vi "Parallel VIs Launcher.vi"() -> ()   [LabVIEW 2013, in "TestVIs.lvlib"]
uses:
  TestVIs.lvlib
panel:
  out "Total Processes Still Running":i16
  out "Total Processes Successfully Launched":i16
  out "Total Processes Requested To Be Launched":i32
  in  "Desired Instances, per kind":i32=2
  # "This will launch a total of 10n + 5 processes"
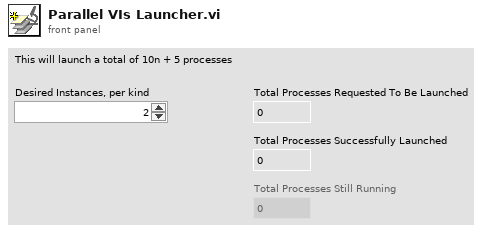
[diagram p1: front panel]
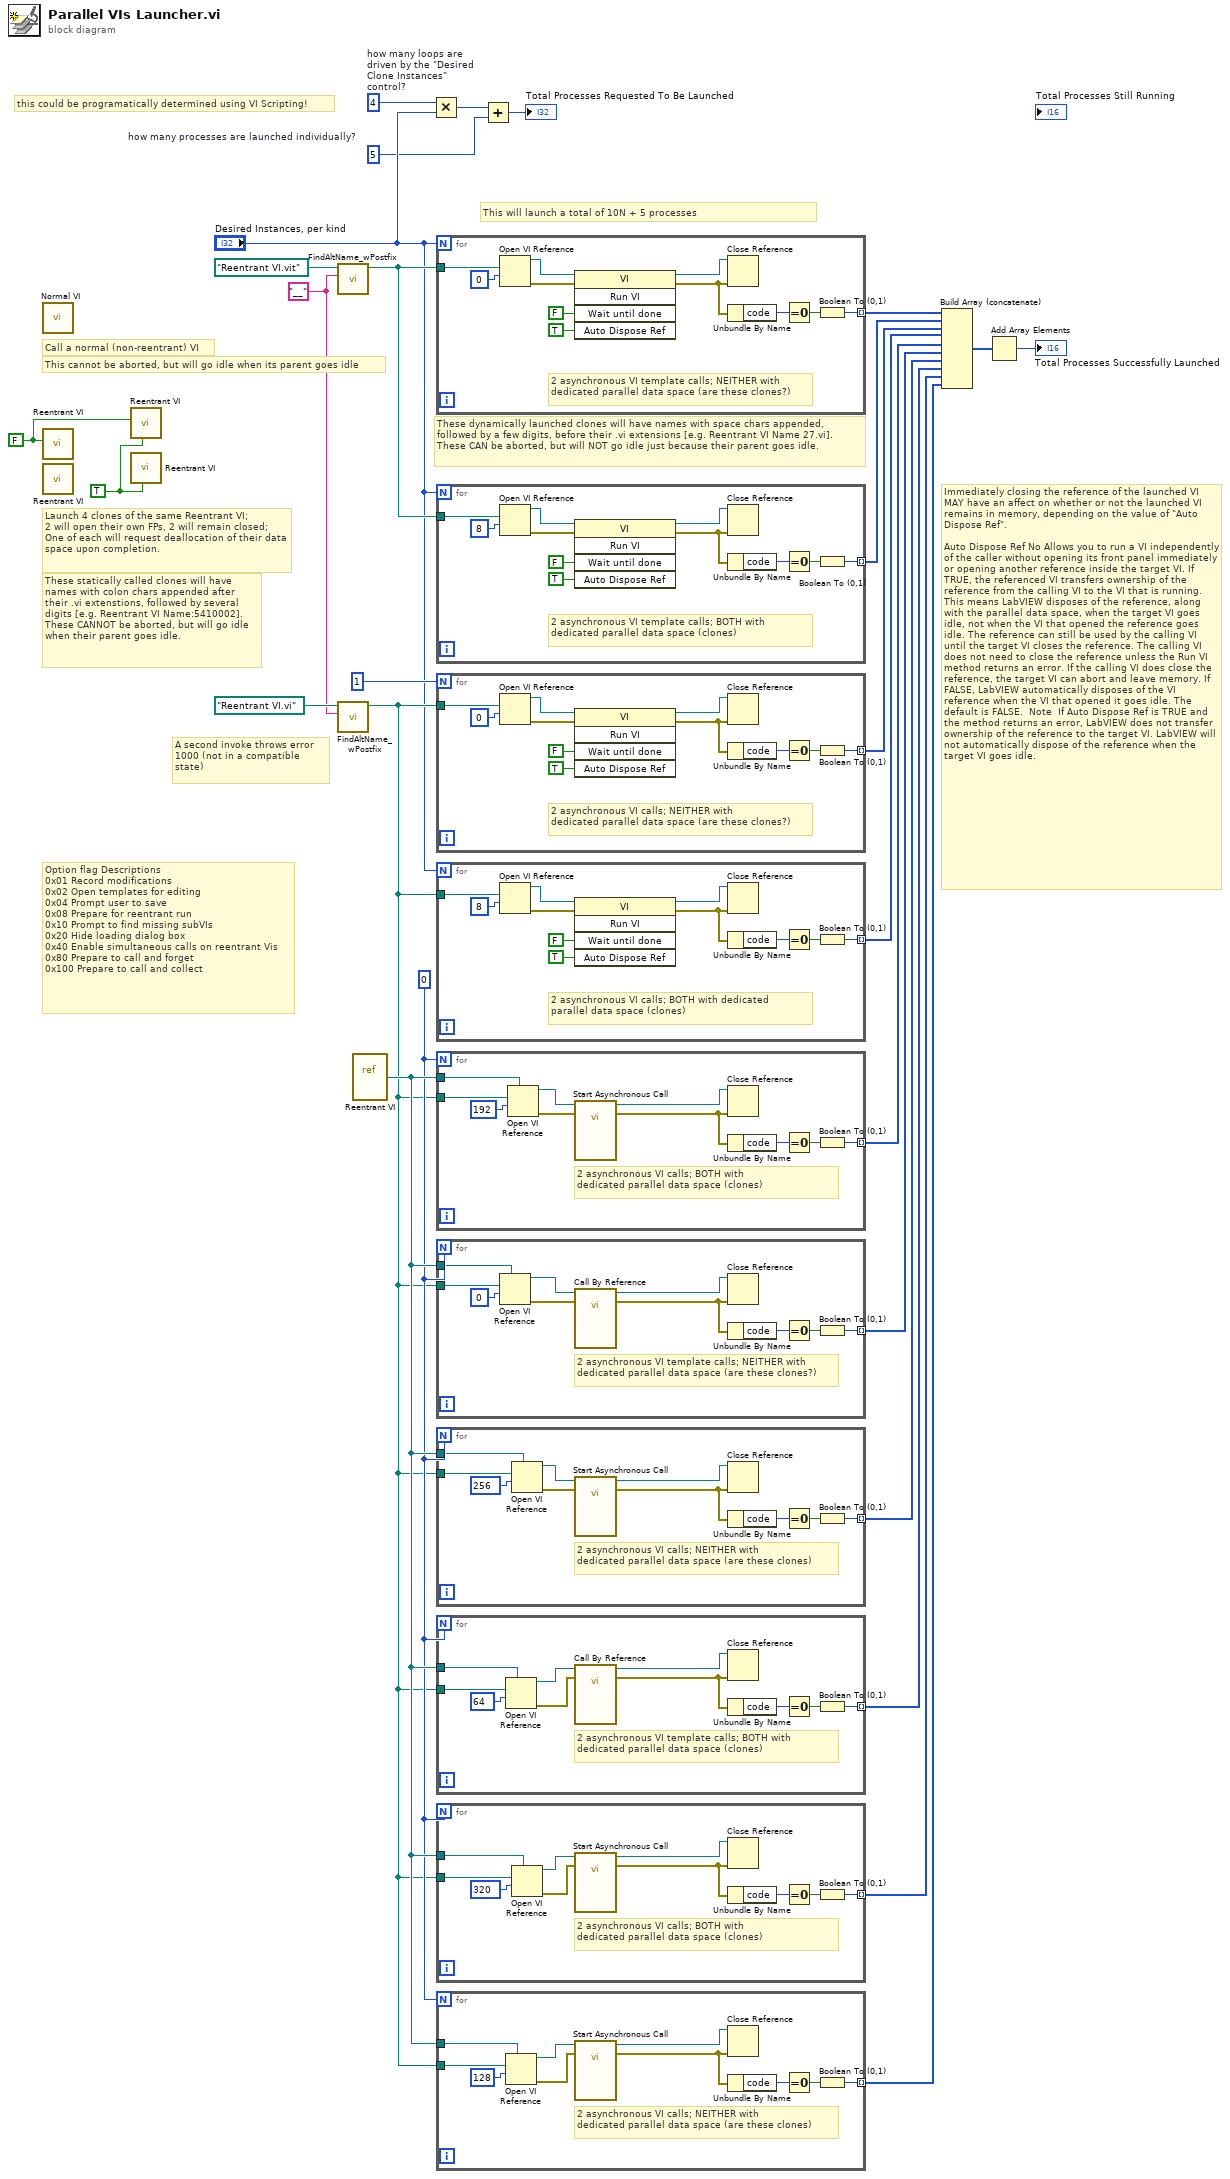
[diagram p0: block diagram]
diagram:
  w14 = 5  # how many processes are launched individually?
  w16 = 4  # how many loops are driven by the "Desired Clone Instances" control?
  w19 = "__" ("Token")
  w23 = 0
  w24 = TRUE ("Request Deallocation?")
  w22 = FALSE ("Open FP?")
  # "Immediately closing the reference of the launched VI MAY have an affect on whether or not the launched VI remains in memory, depending on the value of \"Auto Dispose Ref\".\n\nAuto Dispose Ref No Allows you to run a VI independently of the caller without opening its front panel immediately or opening another reference inside the target VI. If TRUE, the referenced VI transfers ownership of the reference from the calling VI to the VI that is running. This means LabVIEW disposes of the reference, along with the parallel data space, when the target VI goes idle, not when the VI that opened the reference goes idle. The reference can still be used by the calling VI until the target VI closes the reference. The calling VI does not need to close the reference unless the Run VI method returns an error. If the calling VI does close the reference, the target VI can abort and leave memory. If FALSE, LabVIEW automatically disposes of the VI reference when the VI that opened it goes idle. The default is FALSE.  Note  If Auto Dispose Ref is TRUE and the method returns an error, LabVIEW does not transfer ownership of the reference to the target VI. LabVIEW will not automatically dispose of the reference when the target VI goes idle."
  # "A second invoke throws error 1000 (not in a compatible state)"
  # "Option flag Descriptions \n0x01 Record modifications\n0x02 Open templates for editing\n0x04 Prompt user to save\n0x08 Prepare for reentrant run\n0x10 Prompt to find missing subVIs\n0x20 Hide loading dialog box\n0x40 Enable simultaneous calls on reentrant Vis\n0x80 Prepare to call and forget\n0x100 Prepare to call and collect"
  # "this could be programatically determined using VI Scripting!"
  # "These dynamically launched clones will have names with space chars appended, followed by a few digits, before their .vi extensions [e.g. Reentrant VI Name 27.vi].\nThese CAN be aborted, but will NOT go idle just because their parent goes idle."
  # "These statically called clones will have names with colon chars appended after their .vi extenstions, followed by several digits [e.g. Reentrant VI Name:5410002].\nThese CANNOT be aborted, but will go idle when their parent goes idle."
  # "This cannot be aborted, but will go idle when its parent goes idle"
  # "This will launch a total of 10N + 5 processes"
  # "Call a normal (non-reentrant) VI"
  # "Launch 4 clones of the same Reentrant VI; \n2 will open their own FPs, 2 will remain closed; One of each will request deallocation of their data space upon completion."
  n1 = call "Normal VI.vi"() -> ()  [unwired: 12 in]
  n2 = call "Reentrant VI.vi"("Open FP? (T)"=w22) -> ()  [unwired: 11 in]
  n3 = call "Reentrant VI.vi"() -> ()  [unwired: 12 in]
  n4 = call "Reentrant VI.vi"("Request Deallocation?"=w24, "Open FP? (T)"=w22) -> ()  [unwired: 10 in]
  n5 = call "Reentrant VI.vi"("Request Deallocation?"=w24) -> ()  [unwired: 11 in]
  n6 = call "FindAltName_wPostfix.vi"("Token"=w19, "File Path Control in"=path "Reentrant VI.vit" ("vi path")) -> ("File Path Control out"=w21:path)  [unwired: 9 in]
  n7 = call "FindAltName_wPostfix.vi"("Token"=w19, "File Path Control in"=path "Reentrant VI.vi" ("vi path")) -> ("File Path Control out"=w20:path)  [unwired: 9 in]
  n8 = vi-ref "Reentrant VI.vi"() -> (w26:refnum<vi>)
  n9 = Multiply(x=w16, y="Desired Instances, per kind") -> (x*y=w15:i32)
  n10 = for {
    N: "Desired Instances, per kind" -> [_]
    tunnel: w21 -> [w32]
    tunnel: [w28] -> w12 mode=indexing
    # "2 asynchronous VI template calls; NEITHER with \ndedicated parallel data space (are these clones?)"
    n11 = Open VI Reference(vi path=w32, options=0) -> (vi reference=w38:refnum<vi>, error out=w37:errorcluster)  [unwired: 4 in]
    n12 = invoke class="VI" method="Run VI"(reference=w38, error in=w37, "Wait until done"=FALSE ("Wait Until Done"), "Auto Dispose Ref"=TRUE ("Auto Dispose Reference")) -> (reference out=w34:refnum<vi>, error out=w31:errorcluster)  [unwired: 1 in, 3 out]
    n13 = Close Reference(reference=w34, error in (no error)=w31) -> ()  [unwired: 1 out]
    n14 = Unbundle By Name(w31) -> ("code"=w30:i32)
    n15 = Equal To 0?(x=w30) -> (x = 0?=w29:bool)
    n16 = Boolean To (0,1)(Boolean=w29) -> (0, 1=w28:i16)
  }
  n17 = for {
    N: "Desired Instances, per kind" -> [_]
    tunnel: w21 -> [w43]
    tunnel: [w39] -> w9 mode=indexing
    # "2 asynchronous VI template calls; BOTH with \ndedicated parallel data space (clones)"
    n18 = Open VI Reference(vi path=w43, options=8) -> (vi reference=w49:refnum<vi>, error out=w48:errorcluster)  [unwired: 4 in]
    n19 = invoke class="VI" method="Run VI"(reference=w49, error in=w48, "Wait until done"=FALSE ("Wait Until Done"), "Auto Dispose Ref"=TRUE ("Auto Dispose Reference")) -> (reference out=w45:refnum<vi>, error out=w40:errorcluster)  [unwired: 1 in, 3 out]
    n20 = Close Reference(reference=w45, error in (no error)=w40) -> ()  [unwired: 1 out]
    n21 = Unbundle By Name(w40) -> ("code"=w41:i32)
    n22 = Equal To 0?(x=w41) -> (x = 0?=w42:bool)
    n23 = Boolean To (0,1)(Boolean=w42) -> (0, 1=w39:i16)
  }
  n24 = for {
    N: 1 -> [_]
    tunnel: w20 -> [w54]
    tunnel: [w50] -> w8 mode=indexing
    # "2 asynchronous VI calls; NEITHER with \ndedicated parallel data space (are these clones?)"
    n25 = Open VI Reference(vi path=w54, options=0) -> (vi reference=w60:refnum<vi>, error out=w59:errorcluster)  [unwired: 4 in]
    n26 = invoke class="VI" method="Run VI"(reference=w60, error in=w59, "Wait until done"=FALSE ("Wait Until Done"), "Auto Dispose Ref"=TRUE ("Auto Dispose Reference")) -> (reference out=w56:refnum<vi>, error out=w51:errorcluster)  [unwired: 1 in, 3 out]
    n27 = Close Reference(reference=w56, error in (no error)=w51) -> ()  [unwired: 1 out]
    n28 = Unbundle By Name(w51) -> ("code"=w53:i32)
    n29 = Equal To 0?(x=w53) -> (x = 0?=w52:bool)
    n30 = Boolean To (0,1)(Boolean=w52) -> (0, 1=w50:i16)
  }
  n31 = for {
    N: "Desired Instances, per kind" -> [_]
    tunnel: w20 -> [w65]
    tunnel: [w61] -> w7 mode=indexing
    # "2 asynchronous VI calls; BOTH with dedicated \nparallel data space (clones)"
    n32 = Open VI Reference(vi path=w65, options=8) -> (vi reference=w71:refnum<vi>, error out=w70:errorcluster)  [unwired: 4 in]
    n33 = invoke class="VI" method="Run VI"(reference=w71, error in=w70, "Wait until done"=FALSE ("Wait Until Done"), "Auto Dispose Ref"=TRUE ("Auto Dispose Reference")) -> (reference out=w67:refnum<vi>, error out=w62:errorcluster)  [unwired: 1 in, 3 out]
    n34 = Close Reference(reference=w67, error in (no error)=w62) -> ()  [unwired: 1 out]
    n35 = Unbundle By Name(w62) -> ("code"=w63:i32)
    n36 = Equal To 0?(x=w63) -> (x = 0?=w64:bool)
    n37 = Boolean To (0,1)(Boolean=w64) -> (0, 1=w61:i16)
  }
  n38 = for {
    N: w23 -> [_]
    tunnel: w26 -> [w77]
    tunnel: w20 -> [w76]
    tunnel: [w72] -> w6 mode=indexing
    # "2 asynchronous VI calls; BOTH with \ndedicated parallel data space (clones)"
    n39 = Open VI Reference(type specifier VI Refnum (for type only)=w77, vi path=w76, options=192) -> (vi reference=w81:refnum<vi>, error out=w80:errorcluster)  [unwired: 3 in]
    n40 = call-by-ref "Start Asynchronous Call"(reference=w81, error in=w80) -> (reference out=w79:refnum<vi>, error out=w73:errorcluster)  [unwired: 12 in]
    n41 = Close Reference(reference=w79, error in (no error)=w73) -> ()  [unwired: 1 out]
    n42 = Unbundle By Name(w73) -> ("code"=w75:i32)
    n43 = Equal To 0?(x=w75) -> (x = 0?=w74:bool)
    n44 = Boolean To (0,1)(Boolean=w74) -> (0, 1=w72:i16)
  }
  n45 = for {
    N: w23 -> [_]
    tunnel: w26 -> [w87]
    tunnel: w20 -> [w86]
    tunnel: [w82] -> w5 mode=indexing
    # "2 asynchronous VI template calls; NEITHER with \ndedicated parallel data space (are these clones?)"
    n46 = Open VI Reference(type specifier VI Refnum (for type only)=w87, vi path=w86, options=0) -> (vi reference=w91:refnum<vi>, error out=w90:errorcluster)  [unwired: 3 in]
    n47 = call-by-ref "?"(reference=w91, error in=w90) -> (reference out=w89:refnum<vi>, error out=w83:errorcluster)  [unwired: 12 in]
    n48 = Close Reference(reference=w89, error in (no error)=w83) -> ()  [unwired: 1 out]
    n49 = Unbundle By Name(w83) -> ("code"=w84:i32)
    n50 = Equal To 0?(x=w84) -> (x = 0?=w85:bool)
    n51 = Boolean To (0,1)(Boolean=w85) -> (0, 1=w82:i16)
  }
  n52 = for {
    N: w23 -> [_]
    tunnel: w26 -> [w97]
    tunnel: w20 -> [w96]
    tunnel: [w92] -> w4 mode=indexing
    # "2 asynchronous VI calls; NEITHER with \ndedicated parallel data space (are these clones)"
    n53 = Open VI Reference(type specifier VI Refnum (for type only)=w97, vi path=w96, options=256) -> (vi reference=w101:refnum<vi>, error out=w100:errorcluster)  [unwired: 3 in]
    n54 = call-by-ref "Start Asynchronous Call"(reference=w101, error in=w100) -> (reference out=w99:refnum<vi>, error out=w93:errorcluster)  [unwired: 12 in]
    n55 = Close Reference(reference=w99, error in (no error)=w93) -> ()  [unwired: 1 out]
    n56 = Unbundle By Name(w93) -> ("code"=w95:i32)
    n57 = Equal To 0?(x=w95) -> (x = 0?=w94:bool)
    n58 = Boolean To (0,1)(Boolean=w94) -> (0, 1=w92:i16)
  }
  n59 = for {
    N: w23 -> [_]
    tunnel: w26 -> [w107]
    tunnel: w20 -> [w106]
    tunnel: [w102] -> w3 mode=indexing
    # "2 asynchronous VI template calls; BOTH with \ndedicated parallel data space (clones)"
    n60 = Open VI Reference(type specifier VI Refnum (for type only)=w107, vi path=w106, options=64) -> (vi reference=w111:refnum<vi>, error out=w110:errorcluster)  [unwired: 3 in]
    n61 = call-by-ref "?"(reference=w111, error in=w110) -> (reference out=w109:refnum<vi>, error out=w103:errorcluster)  [unwired: 12 in]
    n62 = Close Reference(reference=w109, error in (no error)=w103) -> ()  [unwired: 1 out]
    n63 = Unbundle By Name(w103) -> ("code"=w104:i32)
    n64 = Equal To 0?(x=w104) -> (x = 0?=w105:bool)
    n65 = Boolean To (0,1)(Boolean=w105) -> (0, 1=w102:i16)
  }
  n66 = for {
    N: w23 -> [_]
    tunnel: w26 -> [w117]
    tunnel: w20 -> [w116]
    tunnel: [w112] -> w2 mode=indexing
    # "2 asynchronous VI calls; BOTH with \ndedicated parallel data space (clones)"
    n67 = Open VI Reference(type specifier VI Refnum (for type only)=w117, vi path=w116, options=320) -> (vi reference=w121:refnum<vi>, error out=w120:errorcluster)  [unwired: 3 in]
    n68 = call-by-ref "Start Asynchronous Call"(reference=w121, error in=w120) -> (reference out=w119:refnum<vi>, error out=w113:errorcluster)  [unwired: 12 in]
    n69 = Close Reference(reference=w119, error in (no error)=w113) -> ()  [unwired: 1 out]
    n70 = Unbundle By Name(w113) -> ("code"=w115:i32)
    n71 = Equal To 0?(x=w115) -> (x = 0?=w114:bool)
    n72 = Boolean To (0,1)(Boolean=w114) -> (0, 1=w112:i16)
  }
  n73 = for {
    N: w23 -> [_]
    tunnel: w26 -> [w127]
    tunnel: w20 -> [w126]
    tunnel: [w122] -> w1 mode=indexing
    # "2 asynchronous VI calls; NEITHER with \ndedicated parallel data space (are these clones)"
    n74 = Open VI Reference(type specifier VI Refnum (for type only)=w127, vi path=w126, options=128) -> (vi reference=w131:refnum<vi>, error out=w130:errorcluster)  [unwired: 3 in]
    n75 = call-by-ref "Start Asynchronous Call"(reference=w131, error in=w130) -> (reference out=w129:refnum<vi>, error out=w123:errorcluster)  [unwired: 12 in]
    n76 = Close Reference(reference=w129, error in (no error)=w123) -> ()  [unwired: 1 out]
    n77 = Unbundle By Name(w123) -> ("code"=w124:i32)
    n78 = Equal To 0?(x=w124) -> (x = 0?=w125:bool)
    n79 = Boolean To (0,1)(Boolean=w125) -> (0, 1=w122:i16)
  }
  n80 = Add(x=w15, y=w14) -> (x+y=→"Total Processes Requested To Be Launched":i32)
  n81 = Build Array (concatenate)(w12, w9, w8, w7, w6, w5, w4, w3, w2, w1) -> (w11:i16[])
  n82 = Add Array Elements(numeric array=w11) -> (sum=→"Total Processes Successfully Launched":i16)
